vi "Main.vi"() -> ()   [LabVIEW 2017]
doc: "The myRIO Project template acquires acceleration data from the onboard accelerometer and displays the changes of acceleration values in a waveform chart."
uses:
  <vilib>/myRIO/Common/Instrument Driver Framework/myRIO v1.0/UART/vis/myRIO v1.0 Close UART.vi
  <vilib>/myRIO/Common/Instrument Driver Framework/Utilities/vis/FPGA Ref Manager.vi
  <vilib>/myRIO/Common/Instrument Driver Framework/myRIO v1.0/myRIO v1.0 Reset FPGA.vi
  <vilib>/myRIO/Common/Instrument Driver Framework/myRIO v1.0/IRQ/vis/myRIO v1.0 IRQ Info FGV.vi
  <vilib>/myRIO/Common/Instrument Driver Framework/myRIO v1.0/IRQ/vis/myRIO v1.0 Timer IRQ Info FGV.vi
  <vilib>/myRIO/Common/Instrument Driver Framework/myRIO v1.0/IRQ/vis/myRIO v1.0 ISR Agent.vi
  <vilib>/myRIO/Instrument Drivers/Utilities/Utilities.lvlib
panel:
  out "BUFFER":i32[](array[numeric])
  in  "font file":path
  out "error out":errorcluster
  in  "Stop":bool
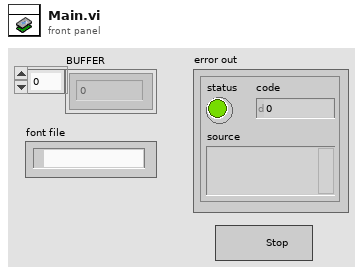
[diagram p1: front panel]
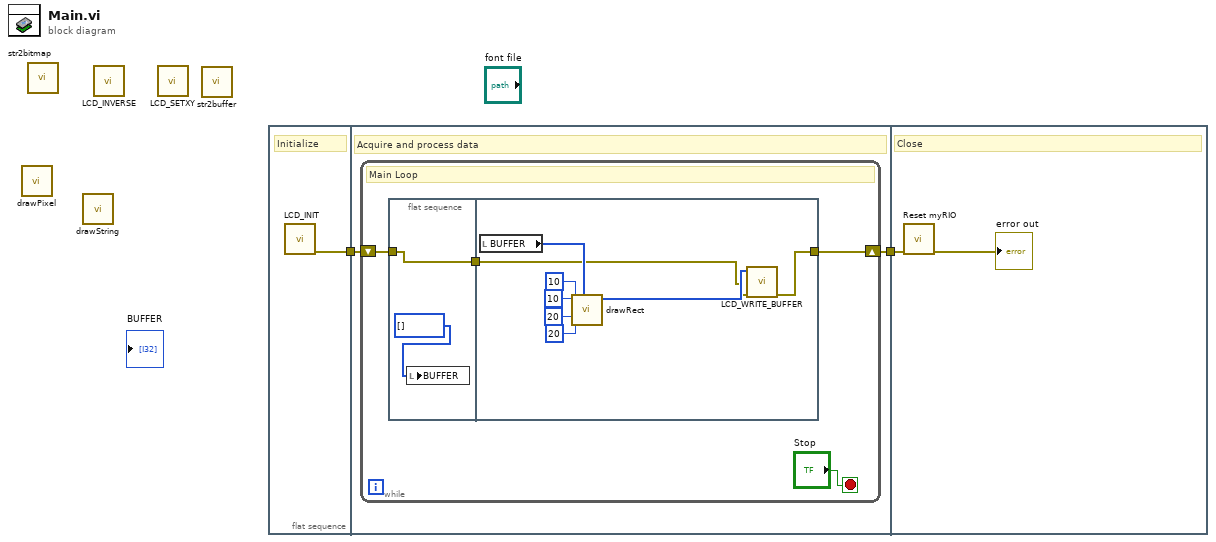
[diagram p0: block diagram]
diagram:
  n1 = call "drawPixel.vi"() -> ()  [unwired: 11 in, 1 out]
  n2 = call "str2bitmap.vi"() -> ()  [unwired: 10 in, 2 out]
  n3 = call "drawString.vi"() -> ()  [unwired: 11 in, 1 out]
  n4 = call "LCD_INVERSE.vi"() -> ()  [unwired: 11 in, 1 out]
  n5 = call "LCD_SETXY.vi"() -> ()  [unwired: 11 in, 1 out]
  n6 = call "str2buffer.vi"() -> ()  [unwired: 9 in, 1 out]
  n7 = flat-sequence {
    tunnel: [w3] -> w2
    tunnel: w2 -> [w5]
    tunnel: [w4] -> w1
    tunnel: w1 -> [w21]
    frame #0 {
      # "Initialize"
      n8 = call "LCD_INIT.vi"() -> ("error out"=w3:errorcluster)  [unwired: 11 in]
    }
    frame #1 {
      # "Acquire and process data"
      n9 = while {
        shift-right: [w8] -> w4
        shift-left: w5 -> [w9]
        stop <- "Stop" stop-if-true
        # "Main Loop"
        n10 = flat-sequence {
          tunnel: w9 -> [w10]
          tunnel: [w10] -> w6
          tunnel: [w19] -> w8
          tunnel: w6 -> [w12]
          frame #0 {
            n11 = local write "BUFFER"(i32[] []) -> ()
          }
          frame #1 {
            n12 = local read "BUFFER"() -> (w14:i32[])
            n13 = call "drawRect.vi"("input_buffer"=w14, "h"=u8 20, "w"=u8 20, "y"=u8 10, "x"=u8 10) -> ("output_buffer"=w13:u8[])  [unwired: 6 in]
            n14 = call "LCD_WRITE_BUFFER.vi"("error in (no error)"=w12, "input_buffer"=w13) -> ("error out"=w19:errorcluster)  [unwired: 9 in]
          }
        }
      }
    }
    frame #2 {
      # "Close"
      n15 = call <vilib>:"Reset myRIO.vi"("error in (no error)"=w21) -> ("error out"=→"error out":errorcluster)  [unwired: 10 in]
    }
  }
